vi "CalculateExtinctionCorrectionsToDoublyChargeParticleContribution.vi"(2 "refractive index, imaginary":sgl=0.1 step=0.01 format="%.3f", 3 "refractive index, real":sgl=1.3 step=0.01 format="%.3f", 4 "Extinction ExtinctionUncertainity Size parameter and Number ofS sizes":T1={"Extinction"=[], "Extinction Uncertainty"=[], "Size parameters"=[], "Number ofSizes"=0.0, "GeometricCrossSection"=[], "Wave Length"=0.0, "SMPS Sizes"=[], "Concentration"=[], "Double Charge Correction"=FALSE, "Extincation Factor"=1.0, "Diameter Factor"=1.0, "Diameter Offset"=0.0, "Extinction Factor Flag"=FALSE, "Diameter Factor Flag"=FALSE, "Diameter Offset Flag"=FALSE, "Sizes"=[], "ExtinctionOrAbsorptionOrScattering"=0, "Concentration(#/cc)"=[]} {"ExtinctionOrAbsorptionOrScattering" scale=0.0..2.0}) -> (0 "Expected Extinction graph":cluster{"Size parameters":dbl[], dbl[]}, 1 "Expected Extinction Cross Section":sgl[](array[numeric]))   [LabVIEW 2013]
uses:
  BaesDataTypeDefinition.ctl
  <vilib>/Analysis/baseanly.llb/Real Dot Product.vi
  <vilib>/imath/engines/lvmath2/RunTimeEngine/ErrorHandling/NIMS_Finalize Error.vi
  <vilib>/imath/engines/lvmath2/RunTimeEngine/Managers/WorkSpace/UID Generator.vi
  <vilib>/imath/engines/lvmath2/RunTimeEngine/Managers/SymbolTable/Clear UID.vi
  <vilib>/imath/engines/lvmath2/RunTimeEngine/NodeEndStatement/NIMS_NodeEndStatement_Output.vi
  <instcachedir>/0/NIMS_NodeEndStatement_Output_53EC0D466D134D7ABD903AC30B43404B.lvgen/NIMS_NodeEndStatement_Output_53EC0D466D134D7ABD903AC30B43404B_005.vi
  <vilib>/imath/engines/lvmath2/RunTimeEngine/RunTimeType/NIMS_RunTimeType_From StrictType (excl LVString).vi
  <instcachedir>/0/NIMS_RunTimeType_From StrictType (excl LVString)_4DEE718D6EB74582AA20236969C084FC.lvgen/NIMS_RunTimeType_From StrictType (excl LVString)_4DEE718D6EB74582AA20236969C084FC_000.vi
  <vilib>/imath/engines/lvmath2/RunTimeEngine/LocalVariableDefStatement/MC_LocalVariableDefStatement_Display.vi
  <instcachedir>/0/NIMS_NodeEndStatement_Output_53EC0D466D134D7ABD903AC30B43404B.lvgen/NIMS_NodeEndStatement_Output_53EC0D466D134D7ABD903AC30B43404B_001.vi
  mie2.dll
  <vilib>/Analysis/NI_AALBase.lvlib
  <vilib>/imath/engines/lvmath2/RunTimeEngine/Managers/SymbolTable/NIMS_WorkSpace.lvlib
panel:
  out "totalscatter 3":sgl=3.7788873
  out "backscatter 3":sgl=8.098428
  out "<cos(theta)> 4":sgl=0.19839454
  out "extinction 3":sgl=1.6240653
  in  "angles (will compute\n2*angles-1 points from\n0...180 degrees)":u32=2
  out "totalscatter 2":sgl=3.7788873
  out "backscatter 2":sgl=8.098428
  out "<cos(theta)> 3":sgl=0.19839454
  out "extinction 2":sgl=1.6240653
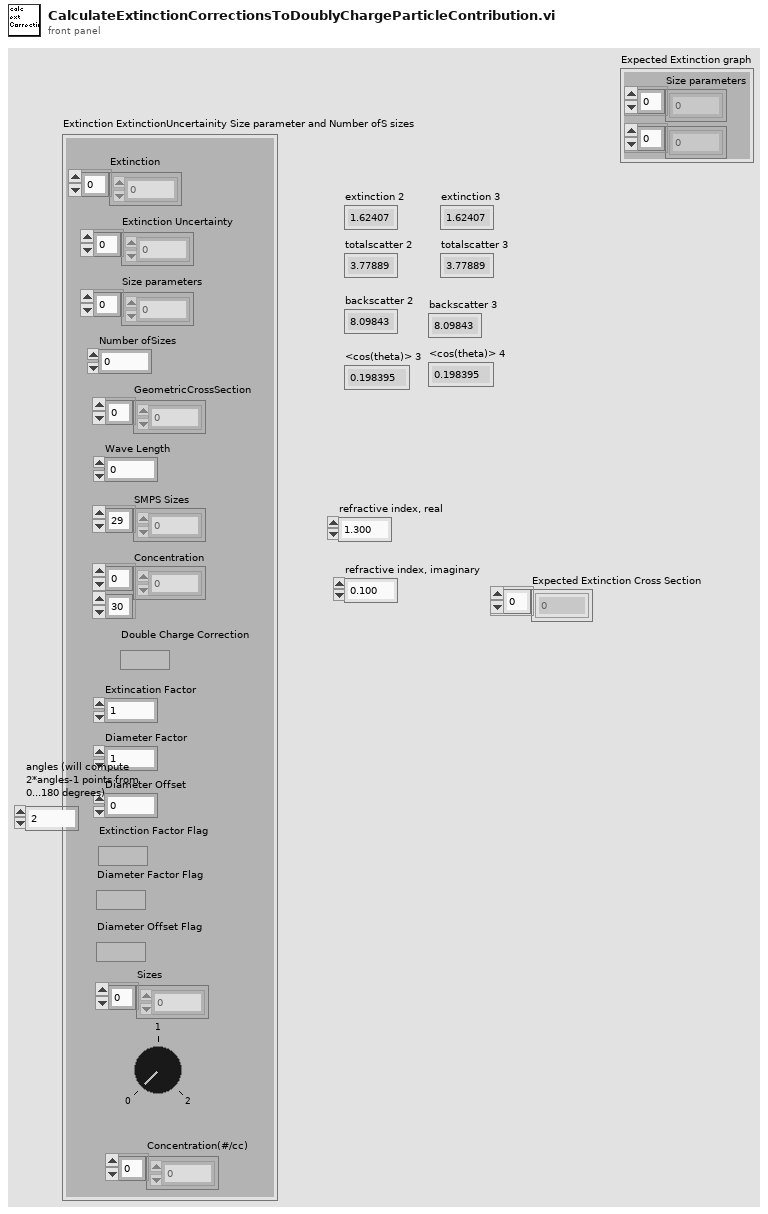
[diagram p1: front panel]
types:
  T1 = typedef "BaesDataTypeDefinition.ctl" = cluster{"Extinction":dbl[], "Extinction Uncertainty":dbl[], "Size parameters":dbl[], "Number ofSizes":dbl, "GeometricCrossSection":dbl[], "Wave Length":dbl, "SMPS Sizes":dbl[], "Concentration":dbl[][], "Double Charge Correction":bool, "Extincation Factor":dbl, "Diameter Factor":dbl, "Diameter Offset":dbl, "Extinction Factor Flag":bool, "Diameter Factor Flag":bool, "Diameter Offset Flag":bool, "Sizes":dbl[], "ExtinctionOrAbsorptionOrScattering":i8, "Concentration(#/cc)":dbl[]}
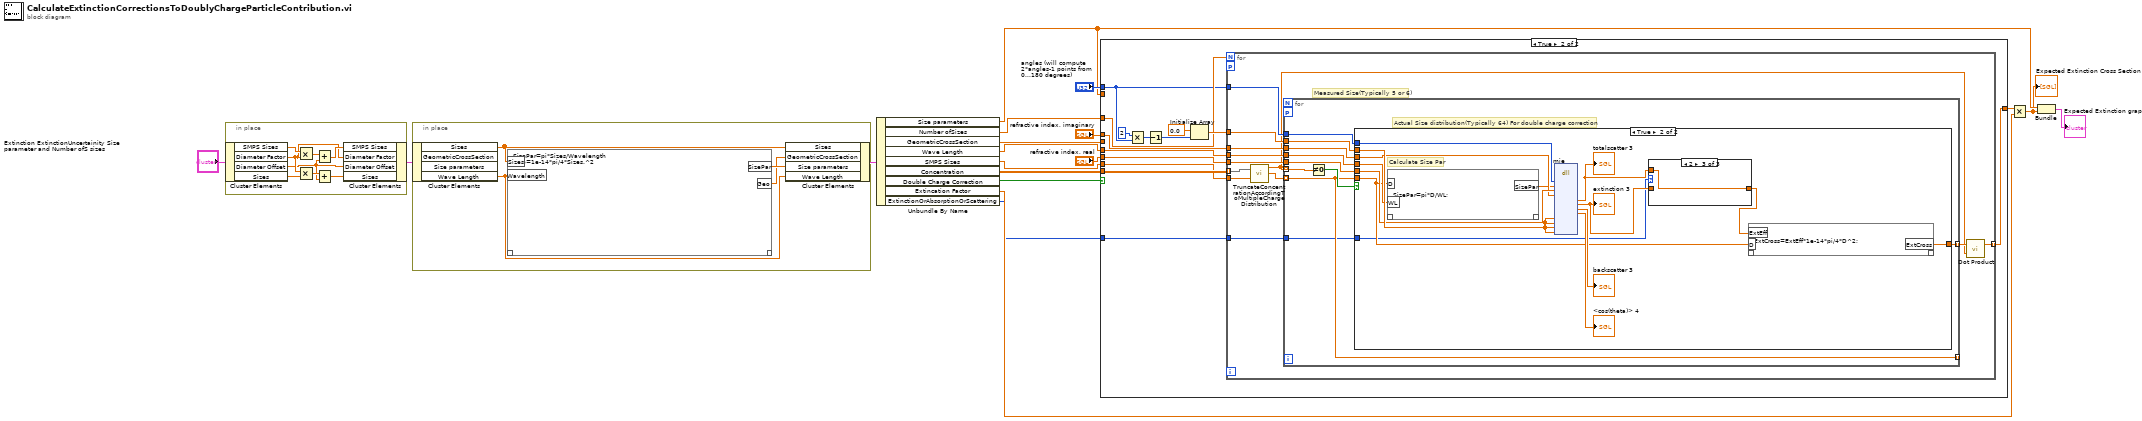
[diagram p0: block diagram]
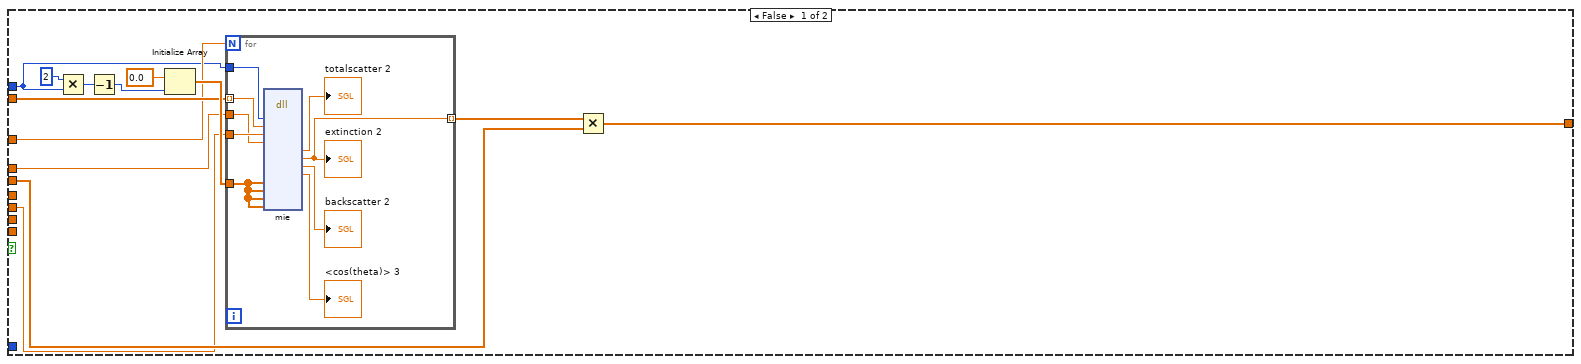
[diagram p2: hidden frame]
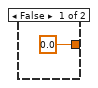
[diagram p3: hidden frame]
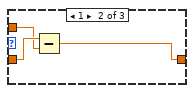
[diagram p5: hidden frame]
diagram:
  n1 = in-place {
    n2 = in-place-cluster #1("Extinction ExtinctionUncertainity Size parameter and Number ofS sizes") -> ("SMPS Sizes"=w26:dbl[], "Diameter Factor"=w22:dbl, "Diameter Offset"=w20:dbl, "Sizes"=w23:dbl[])
    n3 = Multiply(x=w26, y=w22) -> (x*y=w25:dbl[])
    n4 = Multiply(x=w22, y=w23) -> (x*y=w21:dbl[])
    n5 = Add(x=w25, y=w20) -> (x+y=w24:dbl[])
    n6 = Add(x=w21, y=w20) -> (x+y=w19:dbl[])
    n7 = in-place-cluster #1("SMPS Sizes"=w24, "Diameter Factor"=w22, "Diameter Offset"=w20, "Sizes"=w19) -> (w7:T1)
  }
  n8 = in-place {
    n9 = in-place-cluster #2(w7) -> ("Sizes"=w30:dbl[], "Wave Length"=w28:dbl)  [unwired: 2 out]
    n10 = mathscript code="SizePar=pi*Sizes/Wavelength\nGeo=1e-14*pi/4*Sizes.^2"("Sizes"=w30, "Wavelength"=w28) -> ("SizePar"=w29:dbl[], "Geo"=w27:dbl[])  [unwired: 1 in, 1 out]
    n11 = in-place-cluster #2("Sizes"=w30, "GeometricCrossSection"=w27, "Size parameters"=w29, "Wave Length"=w28) -> (w6:T1)
  }
  n12 = Unbundle By Name(w6) -> ("Size parameters"=w11:dbl[], "Number ofSizes"=w18:dbl, "GeometricCrossSection"=w17:dbl[], "Wave Length"=w12:dbl, "SMPS Sizes"=w8:dbl[], "Concentration"=w9:dbl[][], "Double Charge Correction"=w16:bool, "Extincation Factor"=w3:dbl, "ExtinctionOrAbsorptionOrScattering"=w1:i8)
  n13 = case shown="True" w16 {
    tunnel: w11 -> [w99 _]
    tunnel: w18 -> [w98 w122]
    tunnel: w17 -> [w96 _]
    tunnel: "angles (will compute\n2*angles-1 points from\n0...180 degrees)" -> [w95 w121]
    tunnel: "refractive index, imaginary" -> [w94 w120]
    tunnel: "refractive index, real" -> [w93 w119]
    tunnel: w8 -> [_ w115]
    tunnel: w12 -> [_ w118]
    tunnel: w9 -> [_ w116]
    tunnel: [w92 w117] -> w4
    tunnel: w1 -> [_ w114]
    frame False {
      n14 = Multiply(x=u32 2, y=w95) -> (x*y=w103:u32)
      n15 = Decrement(x=w103) -> (x-1=w101:u32)
      n16 = Initialize Array(sgl 0.0, w101) -> (w100:sgl[])
      n17 = for {
        N: w98 -> [_]
        tunnel: w100 -> [w111]
        tunnel: w95 -> [w110]
        tunnel: w93 -> [w109]
        tunnel: w94 -> [w108]
        tunnel: w99 -> [w107] mode=indexing
        tunnel: [w105] -> w97 mode=indexing
        n18 = dll-call lib="Z:/Downloads/Lior Segev Code Projects/RIRetrievalForPASinLabview/mie2.dll" fn="mie"("angles"=w110, "x"=w107, "r"=w109, "i"=w108, "spol_real"=w111, "spol_imaginary"=w111, "ppol_real"=w111, "ppol_imaginary"=w111) -> ("totalscatter"=→"totalscatter 2":sgl, "extinction"=w105:sgl, "backscatter"=→"backscatter 2":sgl, "<cos(theta)>"=→"<cos(theta)> 3":sgl)  [unwired: 16 in, 2 out]
        "extinction 2" <- w105
      }
      n19 = Multiply(x=w97, y=w96) -> (x*y=w92:dbl[])
    }
    frame True {
      n20 = Multiply(x=u32 2, y=w121) -> (x*y=w126:u32)
      n21 = Decrement(x=w126) -> (x-1=w124:u32)
      n22 = Initialize Array(sgl 0.0, w124) -> (w123:sgl[])
      n23 = for {
        N: w122 -> [_]
        tunnel: w123 -> [w139]
        tunnel: w121 -> [w138]
        tunnel: w119 -> [w137]
        tunnel: w120 -> [w136]
        tunnel: w115 -> [w132]
        tunnel: w118 -> [w135]
        tunnel: w116 -> [w130] mode=indexing
        tunnel: [w134] -> w117 mode=indexing
        workers-P: _ -> [_]
        tunnel: w114 -> [w128]
        # "Measured Size(Typically 5 or 6)"
        n24 = call "TruncateConcentrationAccordingToMultipleChargeDistribution.vi"("Concentration"=w130, "Sizes"=w132) -> ("Truncated Concentration"=w129:dbl[], "Truncated Sizes"=w131:dbl[])  [unwired: 1 out]
        n25 = for {
          tunnel: w139 -> [w149]
          tunnel: w138 -> [w148]
          tunnel: w137 -> [w147]
          tunnel: w136 -> [w146]
          tunnel: w131 -> [w141] mode=indexing
          tunnel: w135 -> [w144]
          tunnel: w129 -> [w143] mode=indexing
          tunnel: [w142] -> w133 mode=indexing
          tunnel: [w141] -> _ mode=indexing
          workers-P: _ -> [_]
          tunnel: w128 -> [w140]
          # "Actual Size distribution(Typically 64) For double charge correction"
          n26 = Not Equal To 0?(x=w143) -> (x != 0?=w145:bool)
          n27 = case shown="True" w145 {
            tunnel: w149 -> [_ w162]
            tunnel: w148 -> [_ w161]
            tunnel: w147 -> [_ w160]
            tunnel: w146 -> [_ w159]
            tunnel: w141 -> [_ w157]
            tunnel: w144 -> [_ w158]
            tunnel: [0.0 ("ExtCross") w156] -> w142
            tunnel: w140 -> [_ w151]
            frame False {
            }
            frame True {
              # "Calculate Size Par"
              n28 = mathscript code="SizePar=pi*D/WL;"("D"=w157, "WL"=w158) -> ("SizePar"=w155:dbl)  [unwired: 1 in, 1 out]
              n29 = dll-call lib="Z:/Downloads/Lior Segev Code Projects/RIRetrievalForPASinLabview/mie2.dll" fn="mie"("angles"=w161, "x"=w155, "r"=w160, "i"=w159, "spol_real"=w162, "spol_imaginary"=w162, "ppol_real"=w162, "ppol_imaginary"=w162) -> ("totalscatter"=w152:sgl, "extinction"=w154:sgl, "backscatter"=→"backscatter 3":sgl, "<cos(theta)>"=→"<cos(theta)> 4":sgl)  [unwired: 16 in, 2 out]
              "totalscatter 3" <- w152
              "extinction 3" <- w154
              n30 = case shown="2" w151 {
                tunnel: w154 -> [w165 w168 _]
                tunnel: [w165 w166 w169] -> w153
                tunnel: w152 -> [_ w167 w169]
                frame 0, Default {
                }
                frame 1 {
                  n31 = Subtract(x=w168, y=w167) -> (x-y=w166:sgl)
                }
                frame 2 {
                }
              }
              n32 = mathscript code="ExtCross=ExtEff*1e-14*pi/4*D^2;"("ExtEff"=w153, "D"=w157) -> ("ExtCross"=w156:dbl)  [unwired: 1 in, 1 out]
            }
          }
        }
        n33 = call-poly <vilib>:"Dot Product.vi"("Y Vector"=w129, "X Vector"=w133) -> ("X * Y"=w134:dbl)  [unwired: 1 out]
      }
    }
  }
  n34 = Multiply(x=w4, y=w3) -> (x*y=w2:dbl[])
  "Expected Extinction Cross Section" <- w2
  n35 = Bundle("Size parameters"=w11, w2) -> (→"Expected Extinction graph":cluster{"Size parameters":dbl[], dbl[]})  [unwired: 1 in]
